vi "template VMC.vi"() -> ()   [LabVIEW 2017]
uses:
  Error Handler/Controls/Error Data.ctl
  Error Handler/Controls/Error Type.ctl
  Error Handler/Controls/Error Source.ctl
  Configuration/Controls/Config CMD.ctl
  Configuration/Controls/Config Command.ctl
  Controller/Controls/Controller Overhead.ctl
  Controller/Controls/Controller Transaction.ctl
panel:
  in  "Transaction":refnum<user-event>
  in  "Card Read":refnum<user-event>
  in  "Entered Num":refnum<user-event>
  in  "Overhead DVR":refnum<data-value>
  in  "Funds Dispensed":refnum<user-event>
  in  "Deposit Received":refnum<user-event>
  in  "Config CMD":refnum<user-event>
  in  "Stop DVR":refnum<data-value>
  in  "Stop":refnum<user-event>
  in  "Error":refnum<user-event>
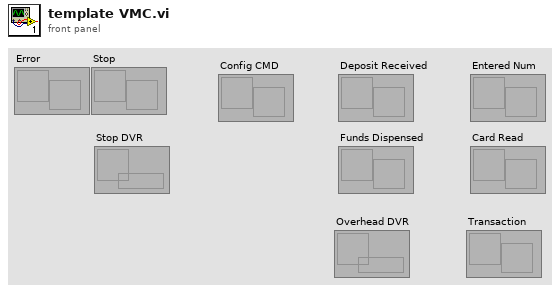
[diagram p1: front panel]
types:
  T1 = typedef "Controller Transaction.ctl" = enum16{"Balance Inquiry", "Deposit", "Withdrawal", "Fast Cash", "New Transaction", "Terminate Session"}
  T2 = typedef "Controller Overhead.ctl" = cluster{"Transaction Message":string, "Message":string, "Card Read":bool, "Account Number":u32, "Amount":u32, "Current Transaction":T1, "Next Transaction":T1}
  T3 = typedef "Config CMD.ctl" = cluster{"CMD":T4, "Data":variant}
  T4 = typedef "Config Command.ctl" = enum16{"Read", "Search", "Update"}
  T5 = typedef "Error Data.ctl" = cluster{"Error Type":T6, "Error Source":T7, "Data":variant}
  T6 = typedef "Error Type.ctl" = enum16{"Console Error", "Sensor Interface IO Error", "Process Step Error"}
  T7 = typedef "Error Source.ctl" = enum16{"User Console", "Display Console", "Sensor Interface"}
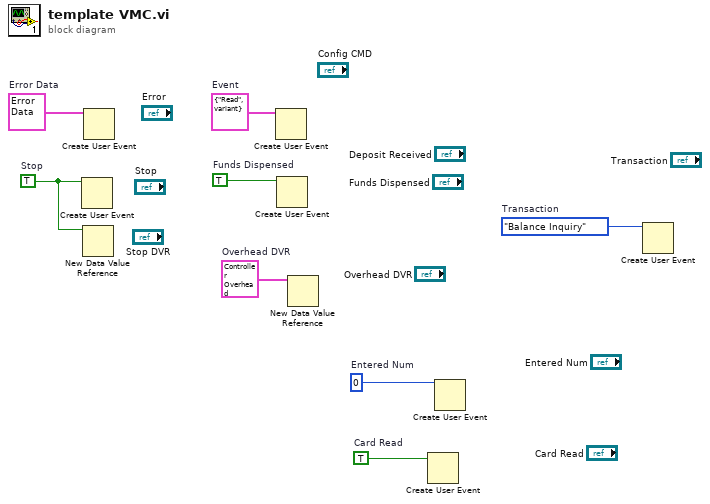
[diagram p0: block diagram]
diagram:
  w1 = Controller_Transaction."Balance Inquiry"  # Transaction
  w2 = TRUE  # Card Read
  w3 = 0  # Entered Num
  w4 = T2 {"Transaction Message"="", "Message"="", "Card Read"=FALSE, "Account Number"=0, "Amount"=0, "Current Transaction"=enum."Balance Inquiry", "Next Transaction"=enum."Balance Inquiry"}  # Overhead DVR
  w5 = TRUE  # Funds Dispensed
  w6 = T3 {"CMD"=enum."Read", "Data"=variant}  # Event
  w7 = TRUE  # Stop
  w8 = T5 {"Error Type"=enum."Console Error", "Error Source"=enum."User Console", "Data"=variant}  # Error Data
  n1 = Create User Event(user event datatype=w7) -> ()  [unwired: 1 in, 2 out]
  n2 = New Data Value Reference(data value=w7) -> ()  [unwired: 1 in, 2 out]
  n3 = Create User Event(user event datatype=w8) -> ()  [unwired: 1 in, 2 out]
  n4 = Create User Event(user event datatype=w6) -> ()  [unwired: 1 in, 2 out]
  n5 = Create User Event(user event datatype=w5) -> ()  [unwired: 1 in, 2 out]
  n6 = New Data Value Reference(data value=w4) -> ()  [unwired: 1 in, 2 out]
  n7 = Create User Event(user event datatype=w2) -> ()  [unwired: 1 in, 2 out]
  n8 = Create User Event(user event datatype=w3) -> ()  [unwired: 1 in, 2 out]
  n9 = Create User Event(user event datatype=w1) -> ()  [unwired: 1 in, 2 out]
